vi "IsModel8743.vi"(8 "error in":errorcluster, 11 "Model / Serial":string) -> (0 "error out":errorcluster, 3 "Boolean":bool)   [LabVIEW 2009]
uses:
  <vilib>/regexp/Match Regular Expression.xnode
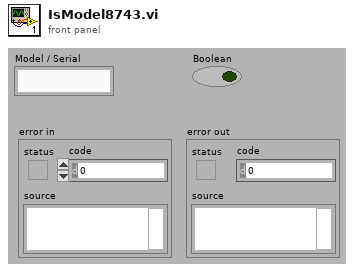
[diagram p1: front panel]
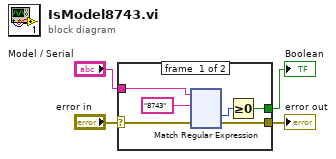
[diagram p0: block diagram]
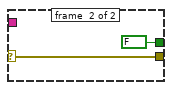
[diagram p2: hidden frame]
diagram:
  n1 = case shown="No Error" "error in" {
    selector: "error in" -> [w5 w119]
    tunnel: [w10 FALSE] -> w4
    tunnel: [w8 w119] -> w3
    tunnel: "Model / Serial" -> [w6 _]
    frame #0 {
      n2 = xnode "Match Regular Expression"("input string"=w6, "regular expression"="8743", "error in"=w5) -> ("offset past match"=w9:i32, "error out"=w8:errorcluster)  [unwired: 3 in, 3 out]
      n3 = Greater Or Equal To 0?(x=w9) -> (x >= 0?=w10:bool)
    }
    frame #1 {
    }
  }
  "Boolean" <- w4
  "error out" <- w3
